vi "CRYFFT Band Filter.vi"(8 "High Freq":dbl=2.0, 9 "Low Freq":dbl=2.0, 10 "Fs":dbl=2.0, 11 "Signal In":dbl[](array[numeric])) -> (3 "Signal out":dbl[](array[numeric]))   [LabVIEW 2013]
uses:
  <vilib>/Analysis/2dsp.llb/Real FFT.vi
  <vilib>/Analysis/2dsp.llb/Inverse Real FFT.vi
  <vilib>/Analysis/NI_AALPro.lvlib
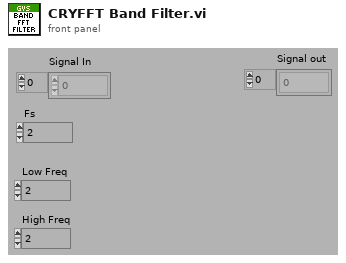
[diagram p1: front panel]
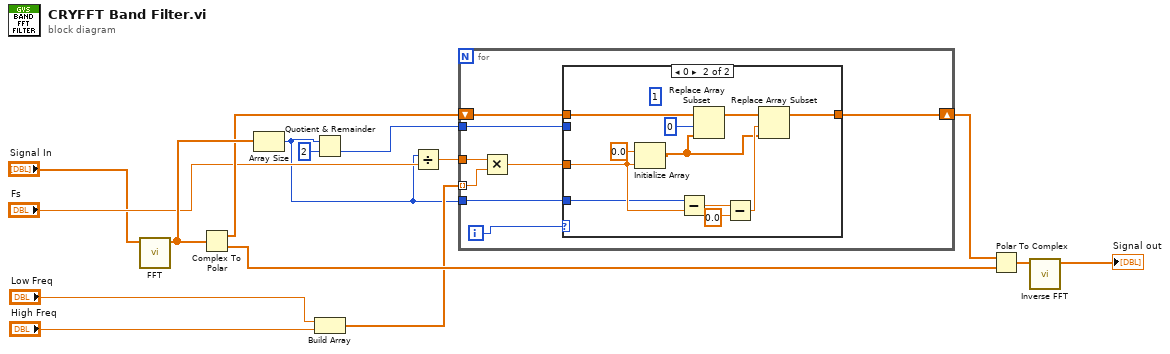
[diagram p0: block diagram]
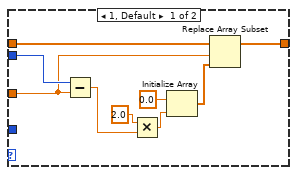
[diagram p2: hidden frame]
diagram:
  n1 = call-poly <vilib>:"FFT.vi"("X"="Signal In") -> ("FFT {X}"=w14:cdb[])  [unwired: 9 in, 1 out]
  n2 = Complex To Polar(r * e^(i*theta)=w14) -> (r=w7:dbl[], theta=w15:dbl[])
  n3 = Array Size(array=w14) -> (size(s)=w2:i32)
  n4 = Quotient & Remainder(x=w2, y=2) -> (floor(x/y)=w8:i32)  [unwired: 1 out]
  n5 = Build Array("Low Freq", "High Freq") -> (w3:dbl[])
  n6 = Divide(x=w2, y="Fs") -> (x/y=w12:dbl)
  n7 = for {
    tunnel: w12 -> [w23]
    shift-right: [w22] -> w5
    shift-left: w7 -> [w21]
    tunnel: w3 -> [w20] mode=indexing
    tunnel: w8 -> [w18]
    tunnel: w2 -> [w16]
    i -> [w19]
    n8 = Multiply(x=w23, y=w20) -> (x*y=w17:dbl)
    n9 = case shown="0" w19 {
      tunnel: [w31 w34] -> w22
      tunnel: w21 -> [w32 w36]
      tunnel: w18 -> [w30 _]
      tunnel: w17 -> [w25 w35]
      tunnel: w16 -> [_ w33]
      frame 1, Default {
        n10 = Subtract(x=w30, y=w25) -> (x-y=w24:dbl)
        n11 = Multiply(x=2.0, y=w24) -> (x*y=w27:dbl)
        n12 = Initialize Array(0.0 ("element"), w27) -> (w26:dbl[])
        n13 = Replace Array Subset(array=w32, new element=w26, index=w25) -> (w31:dbl[])
      }
      frame 0 {
        (unwired) 1 ("index")
        n14 = Initialize Array(0.0 ("element"), w35) -> (w37:dbl[])
        n15 = Subtract(x=w33, y=w35) -> (x-y=w42:dbl)
        n16 = Replace Array Subset(array=w36, new element=w37, index=0) -> (w39:dbl[])
        n17 = Subtract(x=w42, y=0.0) -> (x-y=w40:dbl)
        n18 = Replace Array Subset(array=w39, new element=w37, index=w40) -> (w34:dbl[])
      }
    }
  }
  n19 = Polar To Complex(1:w15, 2:w5) -> (0:w11:cdb[])
  n20 = call-poly <vilib>:"Inverse FFT.vi"("FFT {X}"=w11) -> ("X"=→"Signal out":dbl[])  [unwired: 9 in, 1 out]
